vi "Acquire_Image.vi"(11 "CameraDevRef":T2) -> ()   [LabVIEW 2011]
uses:
  <vilib>/Rock Robotics/WPI/Camera/WPI_CameraDevRef.ctl
  <vilib>/vision/NI_Vision_Development_Module.lvlib
panel:
  out "Number of Particles":i32
  out "Final Binary":T1(plugin-control)
  out "Binary Image":T1(plugin-control)
  out "Green Image":T1(plugin-control)
  out "Rotated Image":T1(plugin-control)
  out "Input Image":T1(plugin-control)
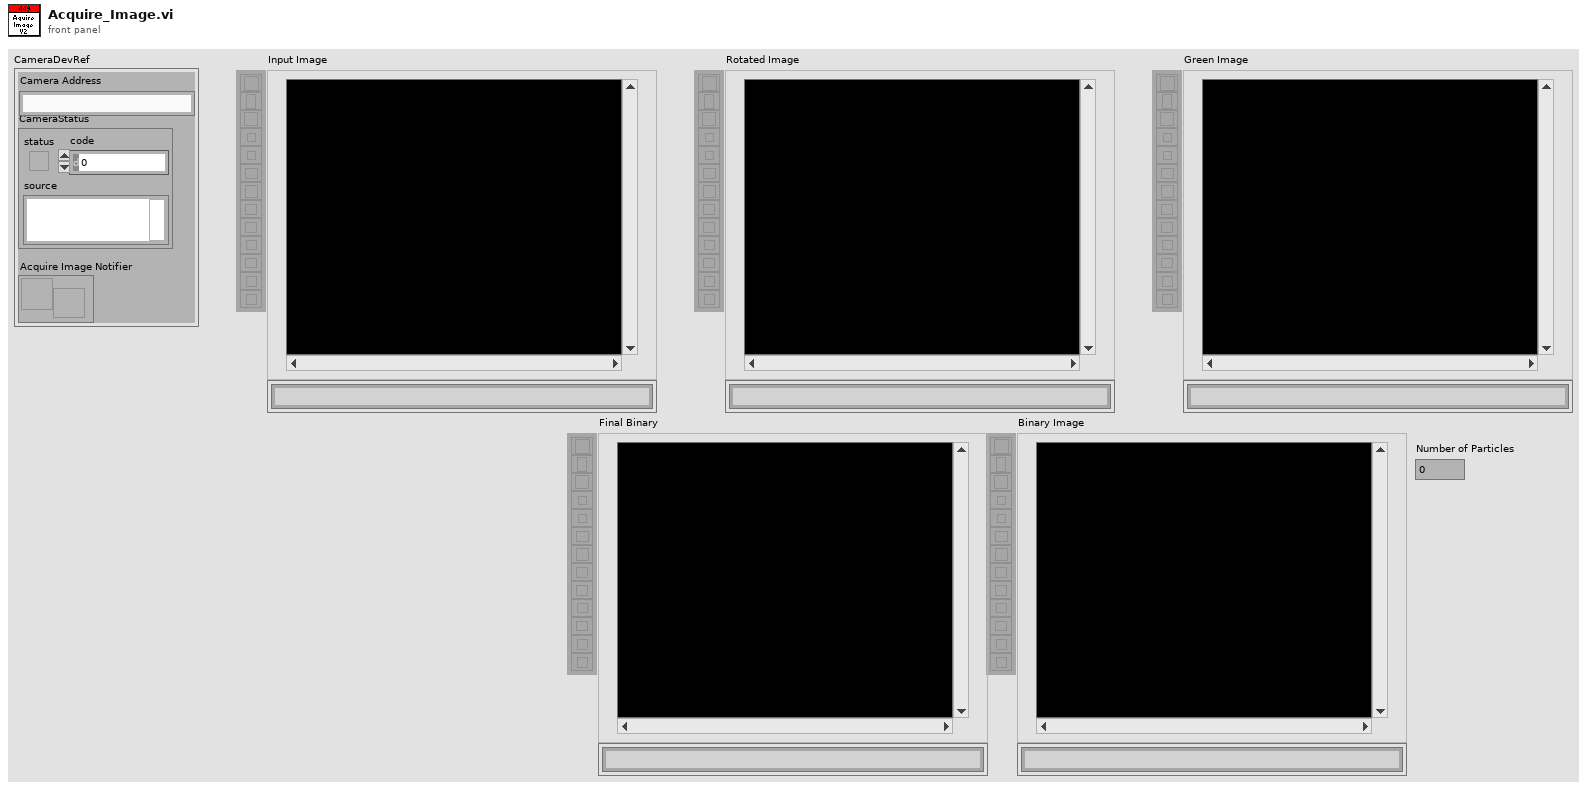
[diagram p1: front panel]
types:
  T1 = typedef "IMAQ Image.ctl" = refnum<image>
  T2 = typedef "WPI_CameraDevRef.ctl" = cluster{"Camera Address":string, "CameraStatus":errorcluster, "Acquire Image Notifier":refnum<notifier>}
  T3 = typedef "Image ClusterV2.ctl" = cluster{"Input Image":T1, "Rotated Image":T1, "Green Image":T1, "Binary Image":T1, "Final Binary":T1, "Horizontal Calibration":T1}
  T4 = enum32{"Differentiation", "Gradient", "Prewitt", "Roberts", "Sigma", "Sobel"}
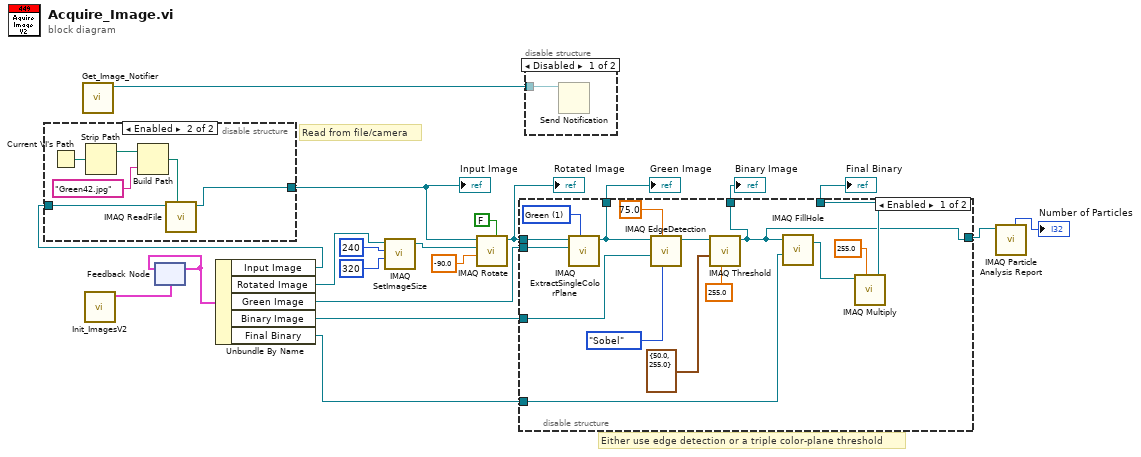
[diagram p0: block diagram]
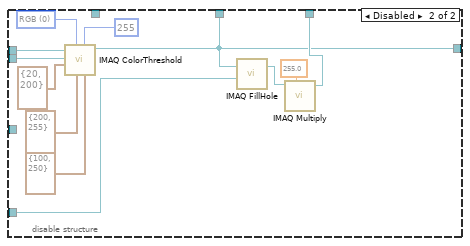
[diagram p2: hidden frame]
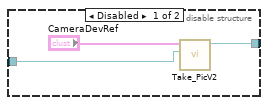
[diagram p4: hidden frame]
diagram:
  # "Either use edge detection or a triple color-plane threshold"
  # "Read from file/camera"
  n1 = call "Get_Image_Notifier.vi"() -> ("notifier out"=w20:refnum<notifier>)  [unwired: 11 in]
  n2 = call "Init_ImagesV2.vi"() -> ("Images"=w19:T3)  [unwired: 11 in]
  n3 = feedback #1(w19) -> (w18:T3)
  n4 = feedback-in #1(w18) -> ()
  n5 = Unbundle By Name(w18) -> ("Input Image"=w17:T1, "Rotated Image"=w11:T1, "Green Image"=w10:T1, "Binary Image"=w6:T1, "Final Binary"=w4:T1)
  n6 = disable-structure shown="Enabled" {
    disable-tunnel: w17 -> [w22 w29]
    disable-tunnel: [w21 w28] -> w9
    frame Disabled {
      n7 = call "Take_PicV2.vi"("Image Src"=w22, "CameraDevRef"="CameraDevRef") -> ("Image Out"=w21:T1)  [unwired: 9 in]
    }
    frame Enabled {
      n8 = Current VI's Path() -> (path=w27:path)
      n9 = Strip Path(path=w27) -> (stripped path=w26:path)  [unwired: 1 out]
      n10 = Build Path(base path=w26, name or relative path="Green42.jpg") -> (appended path=w24:path)
      n11 = call "IMAQ ReadFile"("File Path"=w24, "Image"=w29) -> ("Image Out"=w28:T1)  [unwired: 5 in, 4 out]
    }
  }
  "Input Image" <- w9
  n12 = call "IMAQ SetImageSize"("Y Resolution"=320 ("X Resolution"), "X Resolution"=240 ("Y Resolution"), "Image"=w11) -> ("Image Out"=w12:T1)  [unwired: 2 in, 1 out]
  n13 = call "IMAQ Rotate"("Maintain Size"=FALSE, "Angle (degrees)"=sgl -90.0, "Image Dst"=w12, "Image Src"=w9) -> ("Image Dst Out"=w8:T1)  [unwired: 6 in, 1 out]
  "Rotated Image" <- w8
  n14 = disable-structure shown="Enabled" {
    disable-tunnel: w10 -> [w43 w55]
    disable-tunnel: w8 -> [w42 w56]
    disable-tunnel: [w41 _] -> w7
    disable-tunnel: w6 -> [w40 _]
    disable-tunnel: [w30 w45] -> w5
    disable-tunnel: w4 -> [w34 w49]
    disable-tunnel: [w33 w46] -> w3
    disable-tunnel: [w30 w45] -> w1
    frame Enabled {
      w44 = 1 items=["Red", "Green", "Blue", "Hue", "Saturation", "Luminance", "Value", "Intensity"] ("Color Plane")
      n15 = call "IMAQ ExtractSingleColorPlane"("Color Plane"=w44, "Image Dst"=w43, "Image Src"=w42) -> ("Image Dst Out"=w41:T1)  [unwired: 7 in, 1 out]
      n16 = call "IMAQ EdgeDetection"("Method"=T4."Sobel", "Threshold Value"=sgl 75.0, "Image Dst"=w40, "Image Src"=w41) -> ("Image Dst Out"=w38:T1)  [unwired: 6 in, 1 out]
      n17 = call "IMAQ Threshold"("Replace Value"=sgl 255.0, "Range"=cluster{"Lower value":sgl, "Upper value":sgl} {"Lower value"=50.0, "Upper value"=255.0}, "Image Src"=w38) -> ("Image Dst Out"=w30:T1)  [unwired: 7 in, 1 out]
      n18 = call "IMAQ FillHole"("Image Dst"=w34, "Image Src"=w30) -> ("Image Dst Out"=w31:T1)  [unwired: 4 in, 1 out]
      n19 = call "IMAQ Multiply"("Image Src A"=w31, "Constant"=sgl 255.0) -> ("Image Dst Out"=w33:T1)  [unwired: 5 in, 1 out]
    }
    frame Disabled {
      w52 = u16 0 items=["RGB", "HSL", "HSV", "HSI"] ("Color Mode")
      n20 = call "IMAQ ColorThreshold"("Blue or Luma or Val or Inten Range"=cluster{"Lower value":i32, "Upper value":i32} {"Lower value"=100, "Upper value"=250}, "Replace Value"=255, "Green or Sat Range"=cluster{"Lower value":i32, "Upper value":i32} {"Lower value"=200, "Upper value"=255}, "Color Mode"=w52, "Red or Hue Range"=cluster{"Lower value":i32, "Upper value":i32} {"Lower value"=20, "Upper value"=200}, "Image Dst"=w55, "Image Src"=w56) -> ("Image Dst Out"=w45:T1)  [unwired: 3 in, 1 out]
      n21 = call "IMAQ FillHole"("Image Dst"=w49, "Image Src"=w45) -> ("Image Dst Out"=w48:T1)  [unwired: 4 in, 1 out]
      n22 = call "IMAQ Multiply"("Image Src A"=w48, "Constant"=sgl 255.0) -> ("Image Dst Out"=w46:T1)  [unwired: 5 in, 1 out]
    }
  }
  "Green Image" <- w7
  "Binary Image" <- w5
  "Final Binary" <- w3
  n23 = disable-structure shown="Disabled" {
    disable-tunnel: w20 -> [w57 _]
    frame Disabled {
      n24 = Send Notification(notifier=w57) -> ()  [unwired: 2 in, 2 out]
    }
    frame Enabled {
    }
  }
  n25 = call "IMAQ Particle Analysis Report"("Image"=w1) -> ("Number of Particles"=→"Number of Particles":i32)  [unwired: 5 in, 5 out]
